vi "Fold return code.vi"(7 "command":string, 8 "error in (no error)":errorcluster, 9 "return code":i32) -> (0 "error out":errorcluster)   [LabVIEW 2020, in "NI_WFCN.lvlib"]
doc: "Merges a non-zero process return code (from e.g. System Exec) into error out."
uses:
  <vilib>/net/WFCN/NI_WFCN.lvlib
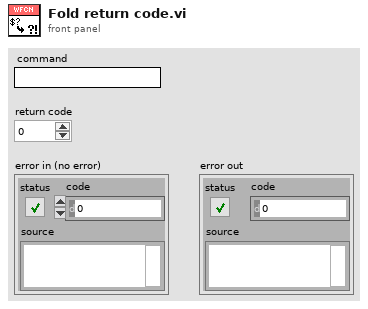
[diagram p1: front panel]
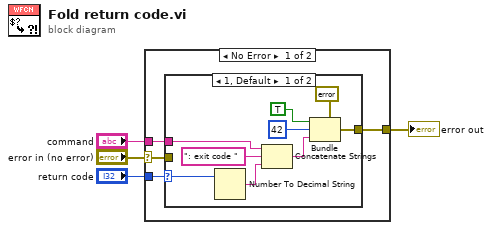
[diagram p0: block diagram]
diagram:
  n1 = case shown="No Error" "error in (no error)" {
    selector: "error in (no error)" -> [w5 w19]
    tunnel: "command" -> [w8 _]
    tunnel: [w7 w19] -> w3
    tunnel: "return code" -> [w6 _]
    frame No Error {
      n2 = case shown="1, Default" w6 {
        selector: w6 -> [w15 _]
        tunnel: w5 -> [_ w18]
        tunnel: w8 -> [w16 _]
        tunnel: [w9 w18] -> w7
        frame 1, Default {
          n3 = Number To Decimal String(number=w15) -> (decimal integer string=w14:string)  [unwired: 1 in]
          n4 = Concatenate Strings(w16, ": exit code " ("format string"), w14) -> (w10:string)
          n5 = Bundle(cluster=errorcluster {"status"=FALSE, "code"=0, "source"=""} ("error out 2"), "status"=TRUE, "code"=42 ("error code (0)"), "source"=w10) -> (w9:errorcluster)
        }
        frame 0 {
        }
      }
    }
    frame Error {
    }
  }
  "error out" <- w3
